vi "test1-AllChainNodesShareTheSameData.vi"(8 "error in (no error)":errorcluster, 11 "TestCase in":refnum<class "testcase-CSMChainMode.lvclass">) -> (0 "error out":errorcluster, 3 "TestCase out":refnum<class "testcase-CSMChainMode.lvclass">)   [LabVIEW 2017, in "testcase-CSMChainMode.lvclass"]
uses:
  testcase-CSMChainMode.lvclass
  src/user.lib/_NEVSTOP/Communicable State Machine(CSM)/_Support/Typedef/_CSM_MODE.ctl
  8deca385-1376-47bb-b92d-c44567c1a462.vi
  <vilib>/addons/_JKI Toolkits/VI Tester/TestCase.llb/TestCase.lvclass
  src/user.lib/_NEVSTOP/Communicable State Machine(CSM)/Communicable State Machine.lvlib
  C:/Program Files (x86)/National Instruments/LabVIEW 2017/vi.lib/addons/_JKI Toolkits/VI Tester/TestCase.llb/TestCase.lvclass
panel:
  out "LoopCount":i32
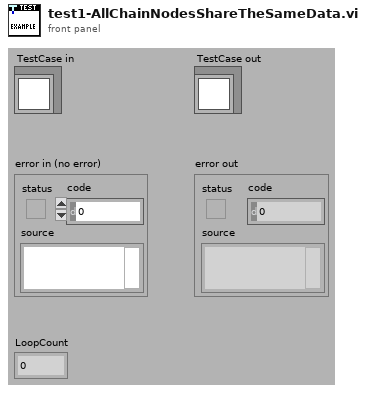
[diagram p1: front panel]
types:
  T1 = typedef "Communicable State Machine.lvlib/_CSM_MODE.ctl" = enum16{"Not Exist", "Stand Alone", "CSM", "Worker", "Worker Agent", "Chain Node", "Chain"}
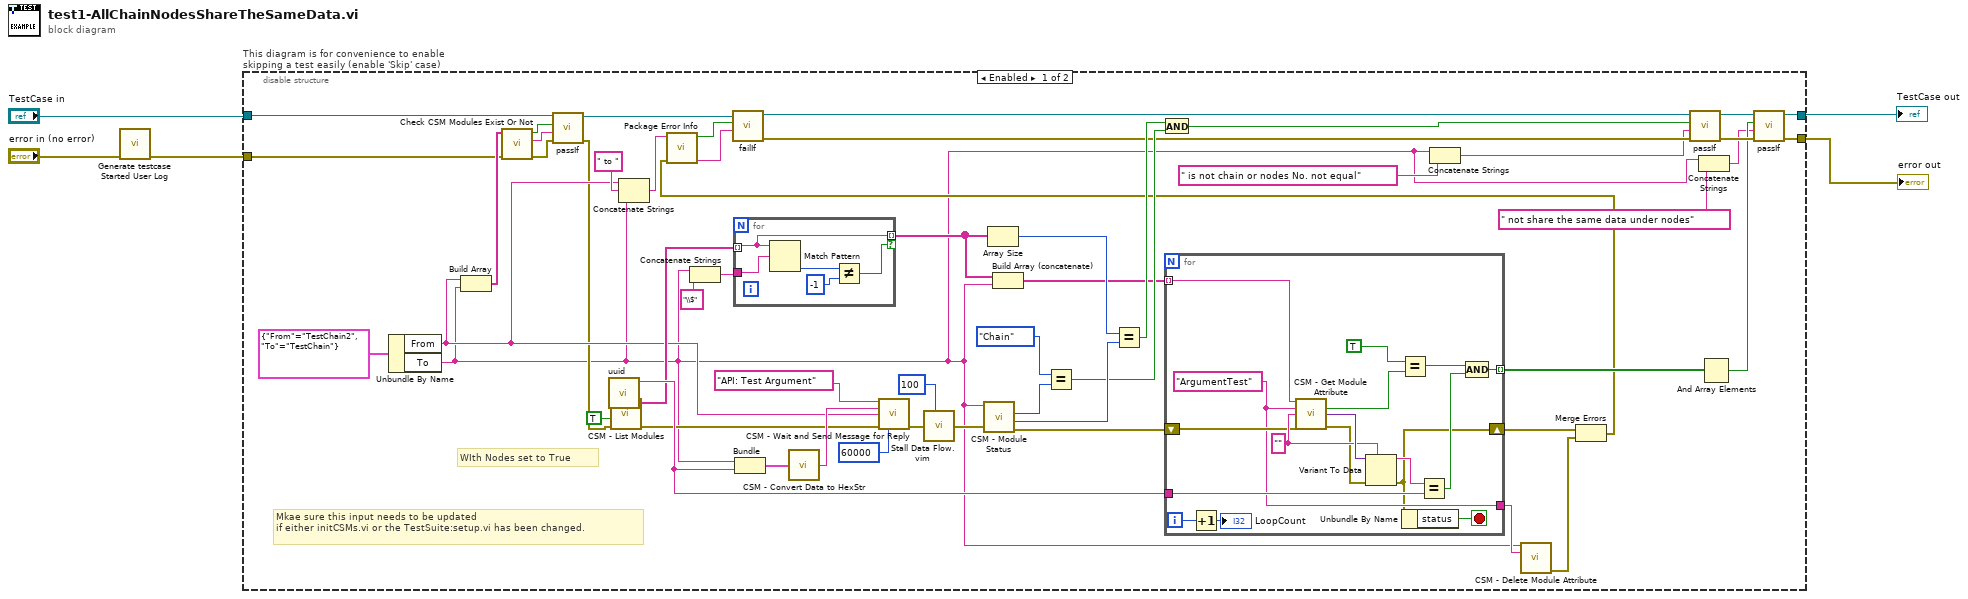
[diagram p0: block diagram]
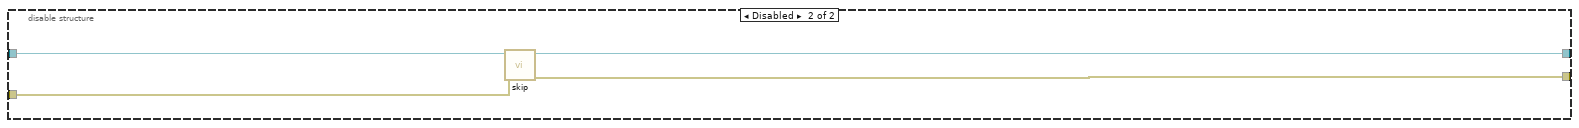
[diagram p2: hidden frame]
diagram:
  n1 = call "Generate testcase Started User Log.vi"("Error In"="error in (no error)") -> ("error out"=w1:errorcluster)  [unwired: 10 in]
  n2 = disable-structure "This diagram is for convenience to enable skipping a test easily (enable 'Skip' case)" shown="Enabled" {
    disable-tunnel: "TestCase in" -> [w15 w85]
    disable-tunnel: [w32 w83] -> w2
    disable-tunnel: [w31 w84] -> w4
    disable-tunnel: w1 -> [w23 w82]
    frame Enabled {
      # "Mkae sure this input needs to be updated \nif either initCSMs.vi or the TestSuite:setup.vi has been changed."
      # "WIth Nodes set to True"
      n3 = Unbundle By Name(cluster{"From":string, "To":string} {"From"="TestChain2", "To"="TestChain"} ("Cluster")) -> ("From"=w18:string, "To"=w8:string)
      n4 = Build Array(w18, w8) -> (w24:string[])
      n5 = call "Check CSM Modules Exist Or Not.vi"("error in"=w23, "CSM names in"=w24) -> ("error out"=w25:errorcluster, "Debug string"=w26:string, "All Modules Exist?"=w27:bool)  [unwired: 7 in]
      n6 = call-dynamic "passIf.vi"("error in (no error)"=w25, "message (\"\")"=w26, "pass"=w27, "TestCase in"=w15) -> ("error out"=w17:errorcluster, "TestCase out"=w14:refnum<class "testcase-CSMChainMode.lvclass">)  [unwired: 6 in]
      n7 = call "uuid.vi"() -> ("UUID"=w54:string)  [unwired: 11 in]
      n8 = call "CSM - List Modules.vi"("Error In"=w17, "With Nodes? (F)"=TRUE) -> ("error out"=w48:errorcluster, "Module Names"=w51:string[])  [unwired: 8 in]
      n9 = Concatenate Strings(w18, " to " ("string"), w8) -> (w19:string)
      n10 = Concatenate Strings(w8, "\\$" ("string")) -> (w29:string)
      n11 = for {
        tunnel: w51 -> [w79] mode=indexing
        tunnel: [w79] -> w40 mode=indexing if=w78
        tunnel: w29 -> [w77]
        n12 = Match Pattern(string=w79, regular expression=w77) -> (offset past match=w81:i32)  [unwired: 1 in, 3 out]
        n13 = Not Equal?(x=w81, y=-1) -> (x != y?=w78:bool)
      }
      n14 = Bundle("To"=w8, "UUID"=w54) -> (w56:cluster{"To":string, "UUID":string})  [unwired: 1 in]
      n15 = call "CSM - Convert Data to HexStr.vi"("Variant"=w56) -> ("HEX String (0-9,A-F)"=w55:string)  [unwired: 8 in]
      n16 = call "CSM - Wait and Send Message for Reply.vi"("State"="API: Test Argument", "Arguments (\"\")"=w55, "Target Module"=w18, "Error In (No Error)"=w48, "Response Timeout (-2 Using Global Settings)"=60000) -> ("error out"=w58:errorcluster)  [unwired: 7 in, 3 out]
      n17 = call "Stall Data Flow.vim"("value in"=w58, "milliseconds to wait"=u32 100) -> ("value out"=w53:errorcluster)  [unwired: 1 out]
      n18 = call "CSM - Module Status.vi"("Error In"=w53, "CSM Name"=w8) -> ("error out"=w38:errorcluster, "#Nodes"=w47:i32, "Mode"=w49:T1)  [unwired: 5 in, 2 out]
      n19 = Array Size(array=w40) -> (size(s)=w46:i32)
      n20 = Build Array (concatenate)(w40, w8) -> (w39:string[])
      n21 = Equal?(x=_CSM_MODE."Chain" ("Mode 2"), y=w49) -> (x = y?=w44:bool)
      n22 = Equal?(x=w46, y=w47) -> (x = y?=w45:bool)
      n23 = And(x=w45, y=w44) -> (x .and. y?=w43:bool)
      n24 = for {
        tunnel: w54 -> [w76]
        tunnel: w39 -> [w67] mode=indexing
        shift-right: [w61] -> w34
        shift-left: w38 -> [w66]
        tunnel: [w65] -> w37 mode=indexing
        tunnel: [w64] -> w35
        i -> [w63]
        stop <- w60 stop-if-true
        w72 = ""
        w64 = "ArgumentTest" ("Attribute")
        n25 = Increment(x=w63) -> (x+1=→"LoopCount":i32)
        n26 = call "CSM - Get Module Attribute.vi"("CSM Name"=w67, "Attribute"=w64, "Default Value (Empty Variant)"=w72, "Error In"=w66) -> ("Found"=w75:bool, "Value"=w73:variant, "error out"=w70:errorcluster)  [unwired: 7 in, 2 out]
        n27 = Variant To Data(error in=w70, type=w72, Variant=w73) -> (data=w71:string, error out=w61:errorcluster)
        n28 = Equal?(x=TRUE, y=w75) -> (x = y?=w69:bool)
        n29 = Unbundle By Name(w61) -> ("status"=w60:bool)
        n30 = Equal?(x=w71, y=w76) -> (x = y?=w68:bool)
        n31 = Compound Arithmetic op=AND(w69, w68) -> (w65:bool)
      }
      n32 = Concatenate Strings(w8, " is not chain or nodes No. not equal" ("string")) -> (w10:string)
      n33 = call "CSM - Delete Module Attribute.vi"("CSM Name"=w8, "Attribute"=w35) -> ("error out"=w33:errorcluster)  [unwired: 10 in, 3 out]
      n34 = Merge Errors(w34, w33) -> (w16:errorcluster)
      n35 = call "Package Error Info.vi"("error in"=w16, "String in"=w19) -> ("packed error info out"=w21:string, "error status"=w22:bool)  [unwired: 8 in]
      n36 = call-dynamic "failIf.vi"("message (\"\")"=w21, "fail"=w22, "TestCase in"=w14) -> ("error out"=w12:errorcluster, "TestCase out"=w13:refnum<class "testcase-CSMChainMode.lvclass">)  [unwired: 7 in]
      n37 = call-dynamic "passIf.vi"("error in (no error)"=w12, "message (\"\")"=w10, "pass"=w43, "TestCase in"=w13) -> ("error out"=w41:errorcluster, "TestCase out"=w42:refnum<class "testcase-CSMChainMode.lvclass">)  [unwired: 6 in]
      n38 = Concatenate Strings(w8, " not share the same data under nodes" ("string")) -> (w7:string)
      n39 = And Array Elements(Boolean array=w37) -> (logical AND=w36:bool)
      n40 = call-dynamic "passIf.vi"("error in (no error)"=w41, "message (\"\")"=w7, "pass"=w36, "TestCase in"=w42) -> ("error out"=w31:errorcluster, "TestCase out"=w32:refnum<class "testcase-CSMChainMode.lvclass">)  [unwired: 6 in]
    }
    frame Disabled {
      # "skip test result while test is under development"
      n41 = call <vilib>:"skip.vi"("error in (no error)"=w82, "TestCase in"=w85) -> ("error out"=w84:errorcluster, "TestCase out"=w83:refnum<class "testcase-CSMChainMode.lvclass">)  [unwired: 8 in]
    }
  }
  "error out" <- w4
  "TestCase out" <- w2
